vi "Psudy emergensy stop.vi"(11 "error In":errorcluster) -> (15 "error out":errorcluster)   [LabVIEW 2011]
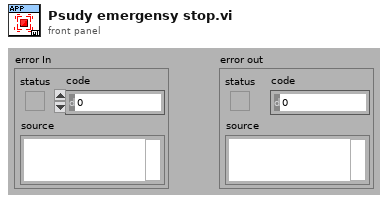
[diagram p1: front panel]
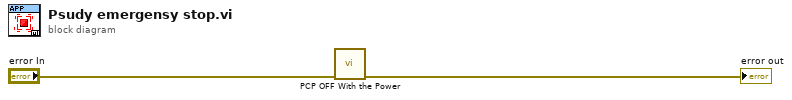
[diagram p0: block diagram]
diagram:
  n1 = call "PCP OFF With the Power.vi"("error In"="error In") -> ("error out"=→"error out":errorcluster)  [unwired: 14 in]
